vi "TextToTextBlocks.vi"(8 "error in (no error)":errorcluster, 11 "string":string) -> (0 "error out":errorcluster, 3 "Blocks":string[](array[string]))   [LabVIEW 2017]
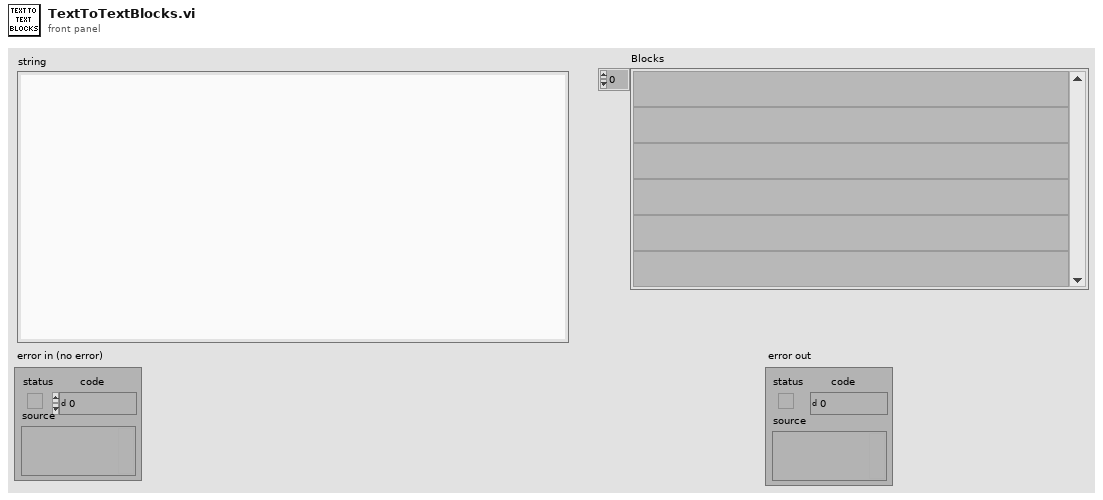
[diagram p1: front panel]
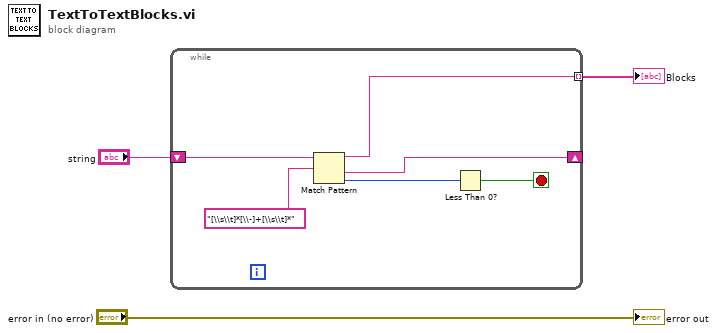
[diagram p0: block diagram]
diagram:
  n1 = while {
    shift-right: [w8] -> _
    shift-left: "string" -> [w9]
    tunnel: [w5] -> w1 mode=indexing
    stop <- w6 stop-if-true
    n2 = Match Pattern(string=w9, regular expression="[\\s\\t]*[\\-]+[\\s\\t]*") -> (before substring=w5:string, after substring=w8:string, offset past match=w7:i32)  [unwired: 1 in, 1 out]
    n3 = Less Than 0?(x=w7) -> (x < 0?=w6:bool)
  }
  "Blocks" <- w1
  "error out" <- "error in (no error)"
